vi "FTW-Image-AppendToPicture.vi"(1 "Image":T1, 3 "Initial Picture":picture) -> (0 "Picture":picture)   [LabVIEW 2013]
doc: "Draws a 1-, 4-, or 8-bit pixmap or a 24-bit RGB pixmap into a picture."
panel:
  # "Inputs"
  # "Outputs"
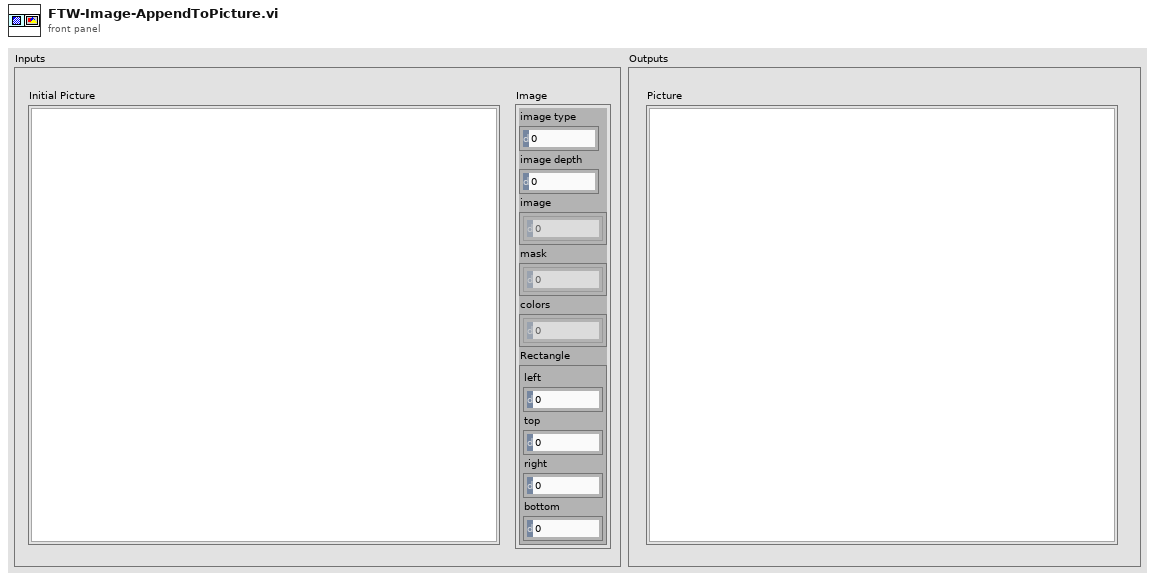
[diagram p1: front panel]
types:
  T1 = cluster{"image type":i32, "image depth":i32, "image":u8[], "mask":u8[], "colors":u32[], "Rectangle":cluster{"left":i16, "top":i16, "right":i16, "bottom":i16}}
  T2 = cluster{"opcode-Copy Pixmap":i16, i32, i32, cluster{"top":i16, "left":i16, i16, i16}, i16, "default foreground":u32, "default background":u32}
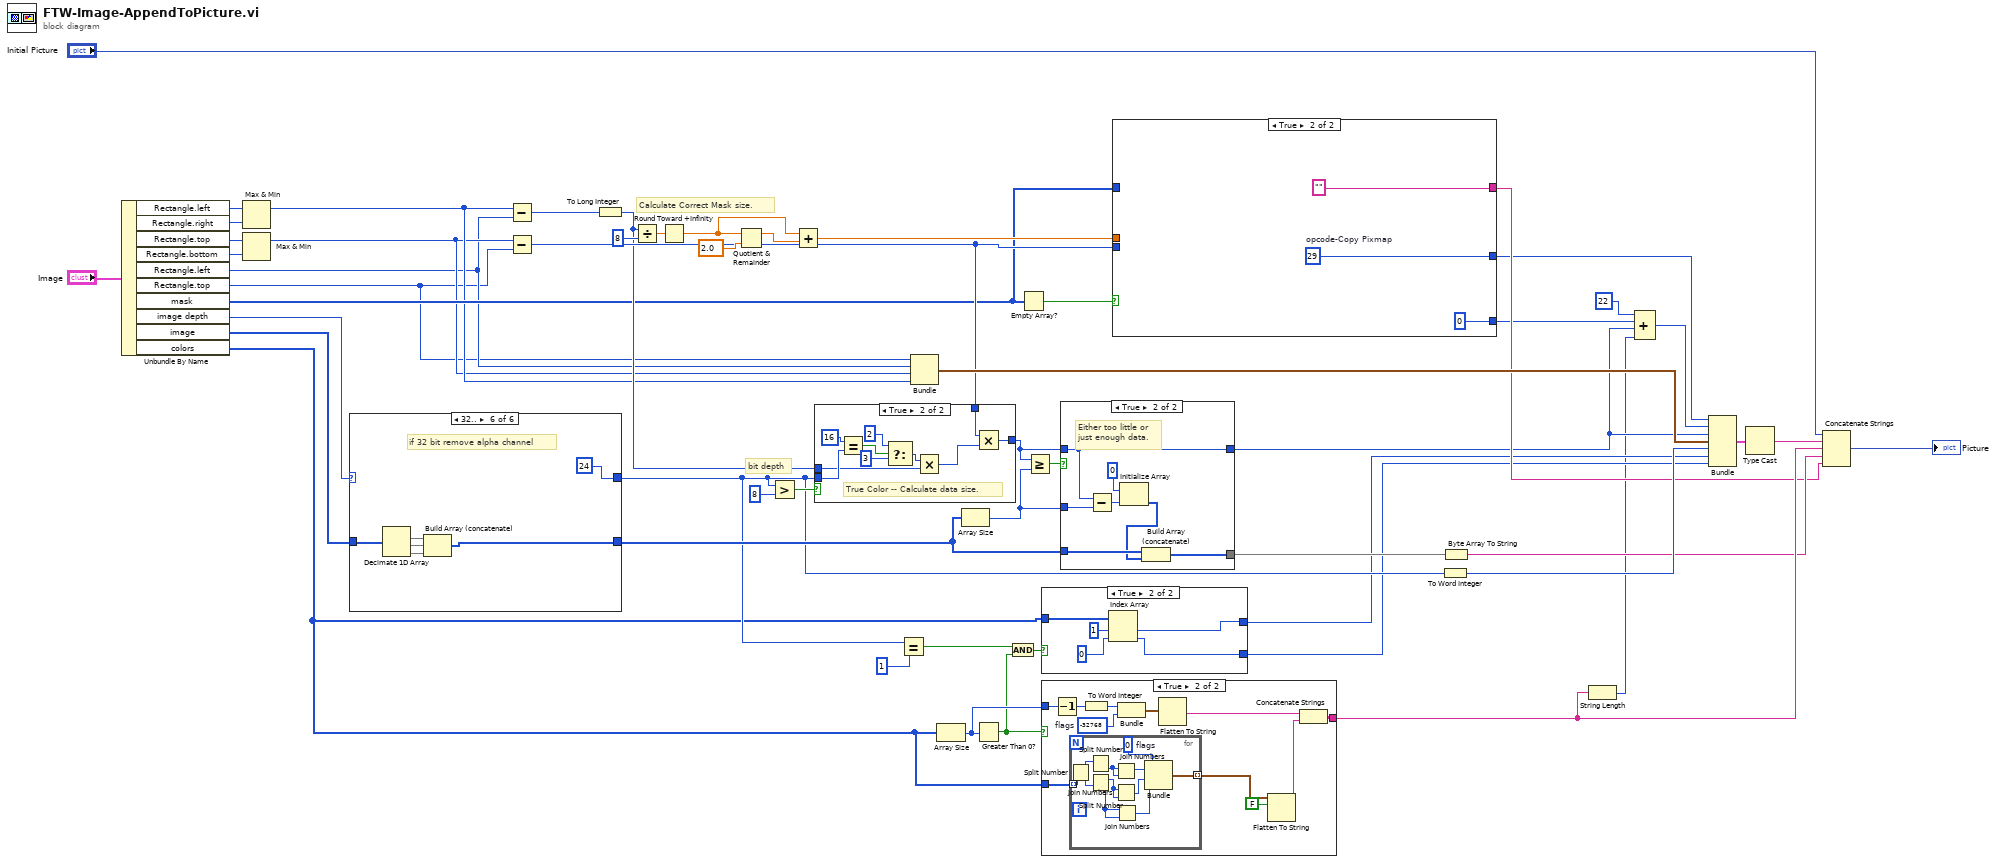
[diagram p0: block diagram]
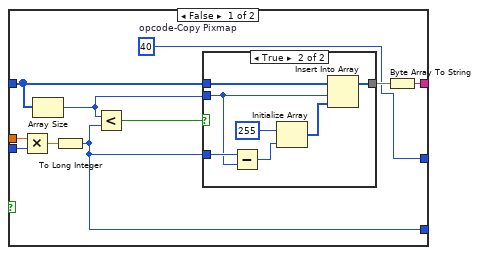
[diagram p2: hidden frame]
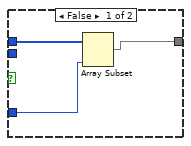
[diagram p3: hidden frame]
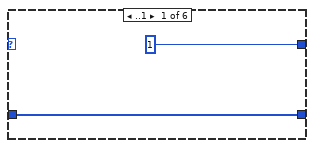
[diagram p4: hidden frame]
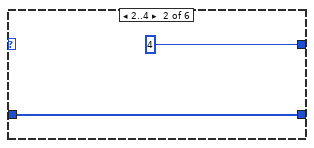
[diagram p5: hidden frame]
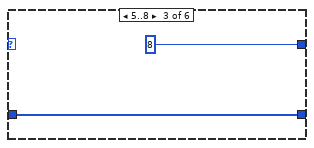
[diagram p6: hidden frame]
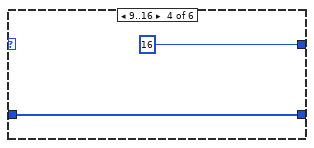
[diagram p7: hidden frame]
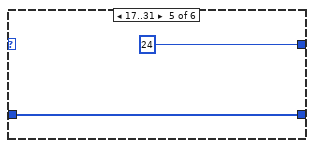
[diagram p8: hidden frame]
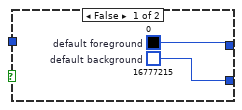
[diagram p9: hidden frame]
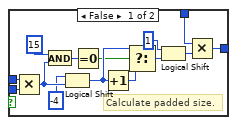
[diagram p10: hidden frame]
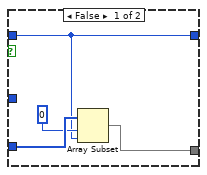
[diagram p11: hidden frame]
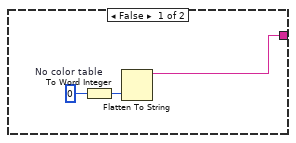
[diagram p12: hidden frame]
diagram:
  # "Calculate Correct Mask size."
  # "bit depth"
  n1 = Unbundle By Name("Image") -> ("Rectangle.left"=w19:i16, "Rectangle.right"=w18:i16, "Rectangle.top"=w17:i16, "Rectangle.bottom"=w16:i16, "Rectangle.left"=w15:i16, "Rectangle.top"=w3:i16, "mask"=w23:u8[], "image depth"=w30:i32, "image"=w29:u8[], "colors"=w2:u32[])
  n2 = Max & Min(x=w19, y=w18) -> (max(x,y)=w21:i16)  [unwired: 1 out]
  n3 = Max & Min(x=w17, y=w16) -> (max(x,y)=w20:i16)  [unwired: 1 out]
  n4 = case shown="32.." w30 {
    tunnel: [1 4 8 16 24 24] -> w22
    tunnel: w29 -> [w55 w57 w59 w61 w63 w68]
    tunnel: [w55 w57 w59 w61 w63 w64] -> w28
    frame ..1 {
    }
    frame 2..4 {
    }
    frame 5..8 {
    }
    frame 9..16 {
    }
    frame 17..31 {
    }
    frame 32.. {
      # "if 32 bit remove alpha channel"
      n5 = Decimate 1D Array(w68) -> (w67:u8[], w66:u8[], w65:u8[])  [unwired: 1 out]
      n6 = Build Array (concatenate)(w67, w66, w65) -> (w64:u8[])
    }
  }
  n7 = Subtract(x=w21, y=w15) -> (x-y=w36:i16)
  n8 = Subtract(x=w20, y=w3) -> (x-y=w33:i16)
  n9 = To Long Integer(number=w36) -> (32bit integer=w31:i32)
  n10 = Divide(x=w31, y=8) -> (x/y=w39:dbl)
  n11 = Round Toward +Infinity(x=w39) -> (ceil(x): smallest int >= x=w38:dbl)
  n12 = Quotient & Remainder(x=w38, y=2.0) -> (x-y*floor(x/y)=w40:dbl)  [unwired: 1 out]
  n13 = Greater?(x=w22, y=8) -> (0:w45:bool)
  n14 = Add(x=w38, y=w40) -> (x+y=w34:dbl)
  n15 = case shown="True" w45 {
    tunnel: [w83 w93] -> w48
    tunnel: w33 -> [w79 w92]
    tunnel: w22 -> [w71 w90]
    tunnel: w31 -> [w70 w88]
    frame False {
      # "Calculate padded size."
      n16 = Multiply(x=w70, y=w71) -> (x*y=w73:i32)
      n17 = And(x=15, y=w73) -> (x .and. y?=w75:i32)
      n18 = Logical Shift(y=-4, x=w73) -> (x << y=w77:i32)
      n19 = Equal To 0?(x=w75) -> (x = 0?=w76:bool)
      n20 = Increment(x=w77) -> (x+1=w78:i32)
      n21 = Select(t=w77, s=w76, f=w78) -> (s? t:f=w81:i32)
      n22 = Logical Shift(y=1, x=w81) -> (x << y=w82:i32)
      n23 = Multiply(x=w79, y=w82) -> (x*y=w83:i32)
    }
    frame True {
      # "True Color -- Calculate data size."
      n24 = Equal?(x=16, y=w90) -> (x = y?=w87:bool)
      n25 = Select(t=2, s=w87, f=3) -> (s? t:f=w84:i32)
      n26 = Multiply(x=w84, y=w88) -> (x*y=w91:i32)
      n27 = Multiply(x=w92, y=w91) -> (x*y=w93:i32)
    }
  }
  n28 = Equal?(x=w22, y=1) -> (x = y?=w42:bool)
  n29 = Bundle("top"=w3, "left"=w15, w20, w21) -> (w35:cluster{"top":i16, "left":i16, i16, i16})  [unwired: 1 in]
  n30 = Array Size(array=w2) -> (size(s)=w53:i32)
  n31 = Array Size(array=w28) -> (size(s)=w47:i32)
  n32 = Greater Than 0?(x=w53) -> (x > 0?=w43:bool)
  n33 = And(x=w42, y=w43) -> (x .and. y?=w44:bool)
  n34 = Empty Array?(array=w23) -> (empty?=w14:bool)
  n35 = Greater Or Equal?(x=w48, y=w47) -> (x >= y?=w49:bool)
  n36 = case shown="True" w44 {
    tunnel: [w95 w98] -> w10
    tunnel: [w94 w96] -> w9
    tunnel: w2 -> [_ w99]
    frame False {
      w94 = u32 16777215  # default background
      w95 = u32 0  # default foreground
    }
    frame True {
      n37 = Index Array(array=w99, index #1=1, index #2=0) -> (element #1=w98:u32, element #2=w96:u32)
    }
  }
  n38 = case shown="True" w43 {
    tunnel: w2 -> [_ w107]
    tunnel: w53 -> [_ w114]
    tunnel: [w101 w109] -> w51
    frame False {
      w103 = 0  # No color table
      n39 = To Word Integer(number=w103) -> (16bit integer=w102:i16)
      n40 = Flatten To String(anything=w102) -> (data string=w101:string)  [unwired: 3 in, 2 out]
    }
    frame True {
      w112 = i16 -32768  # flags
      n41 = Decrement(x=w114) -> (x-1=w108:i32)
      n42 = for {
        tunnel: w107 -> [w123] mode=indexing
        tunnel: [w115] -> w106 mode=indexing
        w122 = i16 0  # flags
        n43 = Split Number(x=w123) -> (hi(x)=w125:u16, lo(x)=w124:u16)
        n44 = Split Number(x=w125) -> (lo(x)=w116:u8)  [unwired: 1 out]
        n45 = Split Number(x=w124) -> (hi(x)=w120:u8, lo(x)=w119:u8)
        n46 = Join Numbers(hi=w116, lo=w116) -> ((hi.lo)=w121:u16)
        n47 = Join Numbers(hi=w120, lo=w120) -> ((hi.lo)=w118:u16)
        n48 = Join Numbers(hi=w119, lo=w119) -> ((hi.lo)=w117:u16)
        n49 = Bundle("flags"=w122, w121, w118, w117) -> (w115:cluster{"flags":i16, u16, u16, u16})  [unwired: 1 in]
      }
      n50 = To Word Integer(number=w108) -> (16bit integer=w113:i16)
      n51 = Bundle(w113, "flags"=w112) -> (w111:cluster{i16, "flags":i16})  [unwired: 1 in]
      n52 = Flatten To String(anything=w111) -> (data string=w110:string)  [unwired: 3 in, 2 out]
      n53 = Flatten To String(anything=w106, prepend array or string size? (T)=FALSE) -> (data string=w104:string)  [unwired: 2 in, 2 out]
      n54 = Concatenate Strings(w110, w104) -> (w109:string)
    }
  }
  n55 = case shown="True" w49 {
    tunnel: w28 -> [w129 w133]
    tunnel: [w128 w134] -> w46
    tunnel: w48 -> [w126 w130]
    tunnel: [w126 w130] -> w6
    tunnel: w47 -> [_ w131]
    frame False {
      n56 = Array Subset(array=w129, index=0, length=w126) -> (w128:u8[])
    }
    frame True {
      # "Either too little or\njust enough data."
      n57 = Subtract(x=w130, y=w131) -> (x-y=w136:i32)
      n58 = Initialize Array(u8 0, w136) -> (w132:u8[])
      n59 = Build Array (concatenate)(w133, w132) -> (w134:u8[])
    }
  }
  n60 = case shown="True" w14 {
    tunnel: w34 -> [w145 _]
    tunnel: w33 -> [w144 _]
    tunnel: [w141 0] -> w7
    tunnel: [w139 ""] -> w32
    tunnel: w23 -> [w138 _]
    tunnel: [w137 w157] -> w13
    frame False {
      w137 = i16 40  # opcode-Copy Pixmap
      n61 = Multiply(x=w145, y=w144) -> (x*y=w146:dbl)
      n62 = Array Size(array=w138) -> (size(s)=w142:i32)
      n63 = To Long Integer(number=w146) -> (32bit integer=w141:i32)
      n64 = Less?(x=w142, y=w141) -> (x < y?=w143:bool)
      n65 = case shown="True" w143 {
        tunnel: w138 -> [w149 w152]
        tunnel: w142 -> [_ w151]
        tunnel: w141 -> [w148 w155]
        tunnel: [w147 w150] -> w140
        frame False {
          n66 = Array Subset(array=w149, length=w148) -> (w147:u8[])  [unwired: 1 in]
        }
        frame True {
          n67 = Subtract(x=w155, y=w151) -> (x-y=w154:i32)
          n68 = Initialize Array(u8 255 ("element"), w154) -> (w153:u8[])
          n69 = Insert Into Array(array=w152, index=w151, new element=w153) -> (w150:u8[])
        }
      }
      n70 = Byte Array To String(unsigned byte array=w140) -> (string=w139:string)
    }
    frame True {
      w157 = i16 29  # opcode-Copy Pixmap
    }
  }
  n71 = To Word Integer(number=w22) -> (16bit integer=w52:i16)
  n72 = Byte Array To String(unsigned byte array=w46) -> (string=w50:string)
  n73 = String Length(string=w51) -> (length=w5:i32)
  n74 = Compound Arithmetic op=ADD(22 ("x"), w7, w6, w5) -> (w4:i32)
  n75 = Bundle("opcode-Copy Pixmap"=w13, w4, w6, w35, w52, "default foreground"=w10, "default background"=w9) -> (w12:T2)  [unwired: 1 in]
  n76 = Type Cast(x=w12) -> (*(type *) &x=w11:string)  [unwired: 1 in]
  n77 = Concatenate Strings("Initial Picture", w11, w51, w50, w32) -> (→"Picture":picture)
